vi "Rotation to Q.vi"(0 "Rotation matrix":T2) -> (1 "quaternion":dbl[](array[numeric]), 2 "theta (rad)":dbl, 3 "axis":dbl[](array[numeric]))   [LabVIEW 2024]
uses:
  <vilib>/Analysis/Matrix/Datatypes/RealMatrix.ctl
  <vilib>/Analysis/Matrix/Datatypes/ComplexMatrix.ctl
  <vilib>/Analysis/_algsub.llb/Real Matrix Trace.vi
  <vilib>/Analysis/_algsub.llb/Real Vector Norm.vi
  <vilib>/Analysis/7linalg.llb/Real Eigenvalues and Vectors.vi
  <vilib>/Analysis/NI_AALPro.lvlib
  <vilib>/Analysis/Matrix/NI_Matrix.lvlib
panel:
  out "norm":dbl
  out "Eigenvalues":cdb[](array[numeric])
  out "Eigenvectors":T1
  # "I have w,x,y,z - python is x,y,z,w"
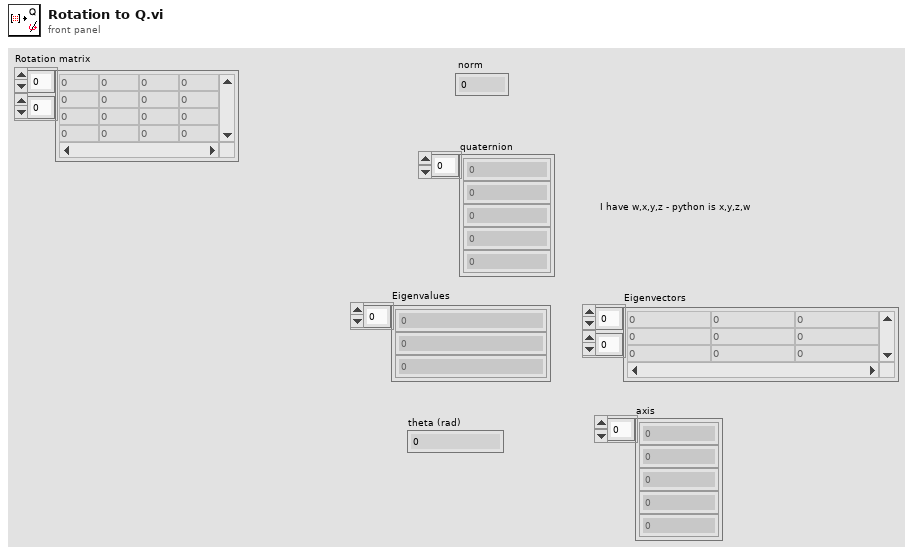
[diagram p1: front panel]
types:
  T1 = typedef "NI_Matrix.lvlib/ComplexMatrix.ctl" = cdb[][]
  T2 = typedef "NI_Matrix.lvlib/RealMatrix.ctl" = dbl[][]
  T3 = enum16{"T>Rii", "R11>R22,R33", "R22>R33", "Rest"}
  T4 = enum16{"T>Rii", "R11>R22,R33", "R22>R33", "Rest"}[]
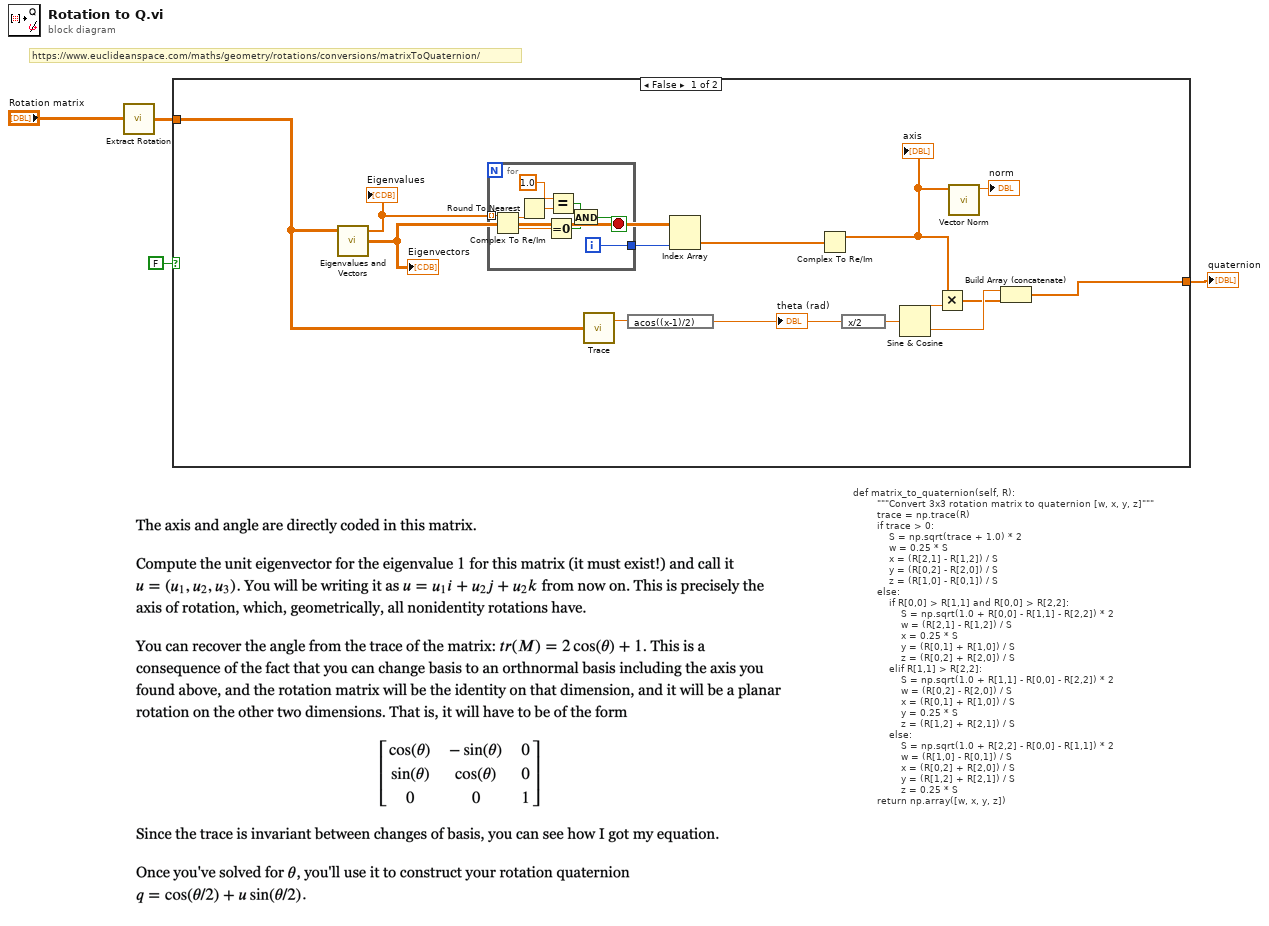
[diagram p0: block diagram]
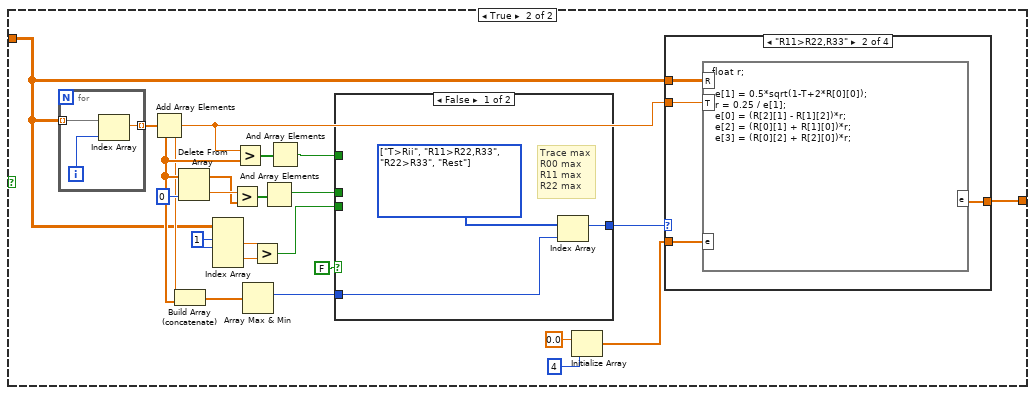
[diagram p2: hidden frame]
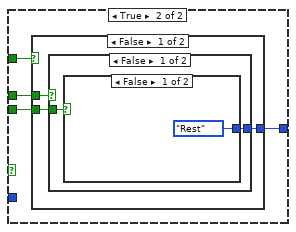
[diagram p3: hidden frame]
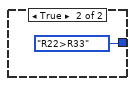
[diagram p4: hidden frame]
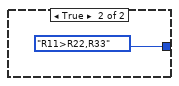
[diagram p5: hidden frame]
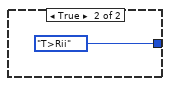
[diagram p6: hidden frame]
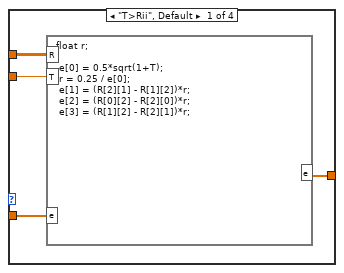
[diagram p7: hidden frame]
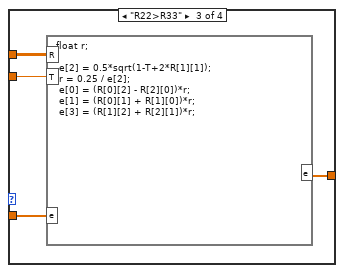
[diagram p8: hidden frame]
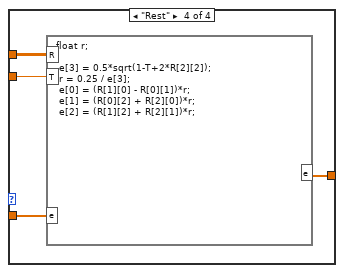
[diagram p9: hidden frame]
diagram:
  # "https://www.euclideanspace.com/maths/geometry/rotations/conversions/matrixToQuaternion/"
  # "def matrix_to_quaternion(self, R):\n        \"\"\"Convert 3x3 rotation matrix to quaternion [w, x, y, z]\"\"\"\n        trace = np.trace(R)\n        if trace > 0:\n            S = np.sqrt(trace + 1.0) * 2\n            w = 0.25 * S\n            x = (R[2,1] - R[1,2]) / S\n            y = (R[0,2] - R[2,0]) / S\n            z = (R[1,0] - R[0,1]) / S\n        else:\n            if R[0,0] > R[1,1] and R[0,0] > R[2,2]:\n                S = np.sqrt(1.0 + R[0,0] - R[1,1] - R[2,2]) * 2\n                w = (R[2,1] - R[1,2]) / S\n                x = 0.25 * S\n                y = (R[0,1] + R[1,0]) / S\n                z = (R[0,2] + R[2,0]) / S\n            elif R[1,1] > R[2,2]:\n                S = np.sqrt(1.0 + R[1,1] - R[0,0] - R[2,2]) * 2\n                w = (R[0,2] - R[2,0]) / S\n                x = (R[0,1] + R[1,0]) / S\n                y = 0.25 * S\n                z = (R[1,2] + R[2,1]) / S\n            else:\n                S = np.sqrt(1.0 + R[2,2] - R[0,0] - R[1,1]) * 2\n                w = (R[1,0] - R[0,1]) / S\n                x = (R[0,2] + R[2,0]) / S\n                y = (R[1,2] + R[2,1]) / S\n                z = 0.25 * S\n        return np.array([w, x, y, z])"
  n1 = call <userlib>:"Extract Rotation.vi"("Transformation matrix"="Rotation matrix") -> ("Rotation matrix"=w2:T2)
  n2 = case shown="False" FALSE {
    tunnel: [w5 w35] -> w4
    tunnel: w2 -> [w6 w28]
    frame False {
      n3 = call-poly <vilib>:"Eigenvalues and Vectors.vi"("Input Matrix"=w6) -> ("Eigenvectors"=w7:T1, "Eigenvalues"=w15:cdb[])  [unwired: 2 in, 1 out]
      "Eigenvectors" <- w7
      "Eigenvalues" <- w15
      n4 = for {
        tunnel: w15 -> [w20] mode=indexing
        tunnel: [w27] -> w16
        i -> [w27]
        stop <- w21 stop-if-true
        n5 = Complex To Re/Im(x + iy=w20) -> (x=w25:dbl, y=w26:dbl)
        n6 = Round To Nearest(number=w25) -> (nearest integer value=w19:dbl)
        n7 = Equal To 0?(x=w26) -> (x = 0?=w22:bool)
        n8 = Equal?(x=1.0, y=w19) -> (x = y?=w23:bool)
        n9 = And(x=w23, y=w22) -> (x .and. y?=w21:bool)
      }
      n10 = call-poly <vilib>:"Trace.vi"("Input Matrix"=w6) -> ("trace"=w8:dbl)  [unwired: 1 out]
      n11 = expression code="acos((x-1)/2)"(w8) -> (w14:dbl)
      "theta (rad)" <- w14
      n12 = Index Array(array=w7, index (col)=w16) -> (element=w11:cdb[])  [unwired: 1 in]
      n13 = Complex To Re/Im(x + iy=w11) -> (x=w17:dbl[])  [unwired: 1 out]
      "axis" <- w17
      n14 = expression code="x/2"(w14) -> (w9:dbl)
      n15 = Sine & Cosine(0:w9) -> (1:w10:dbl, 2:w13:dbl)
      n16 = Multiply(x=w17, y=w10) -> (x*y=w12:dbl[])
      n17 = call-poly <vilib>:"Vector Norm.vi"("Input Vector"=w17) -> ("norm"=→"norm":dbl)  [unwired: 9 in, 1 out]
      n18 = Build Array (concatenate)(w13, w12) -> (w5:dbl[])
    }
    frame True {
      w45 = 1 ("index (row)")
      n19 = for {
        tunnel: w28 -> [w84] mode=indexing
        tunnel: [w82] -> w32 mode=indexing
        i -> [w83]
        n20 = Index Array(array=w84, index=w83) -> (element=w82:dbl)
      }
      n21 = Add Array Elements(numeric array=w32) -> (sum=w31:dbl)
      n22 = Build Array (concatenate)(w31, w32) -> (w30:dbl[])
      n23 = Delete From Array(array=w32, index=0) -> (deleted portion=w43:dbl, array with subset deleted=w42:dbl[])  [unwired: 1 in]
      n24 = Index Array(array=w28, index (row) #1=w45, index (col) #1=w45) -> (element #1=w39:dbl, element #2=w38:dbl)  [unwired: 2 in]
      n25 = Greater?(x=w43, y=w42) -> (0:w41:bool[])
      n26 = Greater?(x=w31, y=w32) -> (0:w49:bool[])
      n27 = Array Max & Min(array=w30) -> (max index (indices)=w29:i32)  [unwired: 3 out]
      n28 = Greater?(x=w39, y=w38) -> (0:w37:bool)
      n29 = And Array Elements(Boolean array=w41) -> (logical AND=w40:bool)
      n30 = And Array Elements(Boolean array=w49) -> (logical AND=w46:bool)
      n31 = case shown="False" FALSE {
        tunnel: w46 -> [_ w56]
        tunnel: w40 -> [_ w55]
        tunnel: w37 -> [_ w54]
        tunnel: [w50 w53] -> w34
        tunnel: w29 -> [w51 _]
        frame False {
          w52 = T4 [enum."T>Rii", enum."R11>R22,R33", enum."R22>R33", enum."Rest"] items=["T>Rii", "R11>R22,R33", "R22>R33", "Rest"]
          # "Trace max\nR00 max\nR11 max\nR22 max"
          n32 = Index Array(array=w52, index=w51) -> (element=w50:T3)
        }
        frame True {
          n33 = case shown="False" w56 {
            tunnel: [w58 T3."T>Rii"] -> w53
            tunnel: w55 -> [w59 _]
            tunnel: w54 -> [w57 _]
            frame False {
              n34 = case shown="False" w59 {
                tunnel: [w60 T3."R11>R22,R33"] -> w58
                tunnel: w57 -> [w61 _]
                frame False {
                  n35 = case shown="False" w61 {
                    tunnel: [T3."Rest" T3."R22>R33"] -> w60
                    frame False {
                    }
                    frame True {
                    }
                  }
                }
                frame True {
                }
              }
            }
            frame True {
            }
          }
        }
      }
      n36 = Initialize Array(0.0 ("element"), 4 ("dimension size")) -> (w36:dbl[])
      n37 = case shown="\"R11>R22,R33\"" w34 {
        tunnel: w28 -> [w69 w73 w77 w81]
        tunnel: w31 -> [w68 w72 w76 w80]
        tunnel: w36 -> [w67 w71 w75 w79]
        tunnel: [w66 w70 w74 w78] -> w35
        frame "T>Rii", Default {
          n38 = formula code="float r;\n\n e[0] = 0.5*sqrt(1+T);\n r = 0.25 / e[0];\n e[1] = (R[2][1] - R[1][2])*r;\n e[2] = (R[0][2] - R[2][0])*r;\n e[3] = (R[1][2] - R[2][1])*r;"("R"=w69, "T"=w68, "e"=w67) -> ("e"=w66:dbl[])
        }
        frame "R11>R22,R33" {
          n39 = formula code="float r;\n\n e[1] = 0.5*sqrt(1-T+2*R[0][0]);\n r = 0.25 / e[1];\n e[0] = (R[2][1] - R[1][2])*r;\n e[2] = (R[0][1] + R[1][0])*r;\n e[3] = (R[0][2] + R[2][0])*r;"("R"=w73, "T"=w72, "e"=w71) -> ("e"=w70:dbl[])
        }
        frame "R22>R33" {
          n40 = formula code="float r;\n\n e[2] = 0.5*sqrt(1-T+2*R[1][1]);\n r = 0.25 / e[2];\n e[0] = (R[0][2] - R[2][0])*r;\n e[1] = (R[0][1] + R[1][0])*r;\n e[3] = (R[1][2] + R[2][1])*r;"("R"=w77, "T"=w76, "e"=w75) -> ("e"=w74:dbl[])
        }
        frame "Rest" {
          n41 = formula code="float r;\n\n e[3] = 0.5*sqrt(1-T+2*R[2][2]);\n r = 0.25 / e[3];\n e[0] = (R[1][0] - R[0][1])*r;\n e[1] = (R[0][2] + R[2][0])*r;\n e[2] = (R[1][2] + R[2][1])*r;"("R"=w81, "T"=w80, "e"=w79) -> ("e"=w78:dbl[])
        }
      }
    }
  }
  "quaternion" <- w4
